vi "MAIN_init_all_global.vi"(1 "error in":errorcluster) -> (0 "error out":errorcluster)   [LabVIEW 2015]
uses:
  GLOBAL/Global_MAIN.vi
  GLOBAL/Global_CAMERA.vi
  GLOBAL/Global_MCL_piezo.vi
  GLOBAL/Global_DAQ.vi
  GLOBAL/Global_ASI_stage.vi
  GLOBAL/Global_ABORT.vi
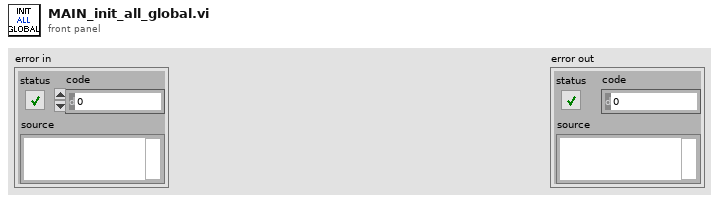
[diagram p1: front panel]
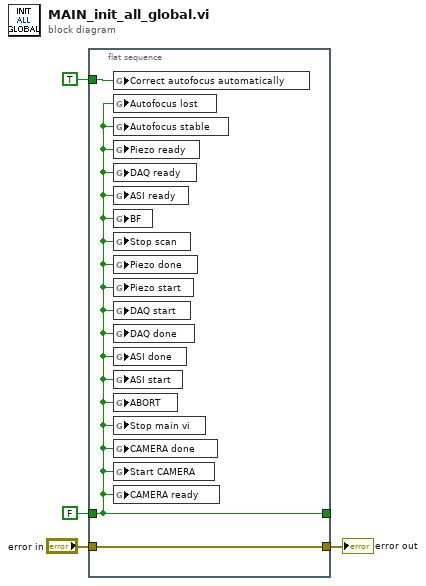
[diagram p0: block diagram]
diagram:
  n1 = flat-sequence {
    tunnel: FALSE ("Stop main vi") -> [w7]
    tunnel: [w7] -> _
    tunnel: "error in" -> [w6]
    tunnel: [w6] -> w2
    tunnel: TRUE ("Stop main vi") -> [w5]
    frame #0 {
      n2 = global write "Global_MAIN.vi" "Correct autofocus automatically"(w5) -> ()
      n3 = global write "Global_MCL_piezo.vi" "Autofocus lost"(w7) -> ()
      n4 = global write "Global_MCL_piezo.vi" "Autofocus stable"(w7) -> ()
      n5 = global write "Global_MCL_piezo.vi" "Piezo ready"(w7) -> ()
      n6 = global write "Global_DAQ.vi" "DAQ ready"(w7) -> ()
      n7 = global write "Global_ASI_stage.vi" "ASI ready"(w7) -> ()
      n8 = global write "Global_ASI_stage.vi" "BF"(w7) -> ()
      n9 = global write "Global_MAIN.vi" "Stop scan"(w7) -> ()
      n10 = global write "Global_MCL_piezo.vi" "Piezo done"(w7) -> ()
      n11 = global write "Global_MCL_piezo.vi" "Piezo start"(w7) -> ()
      n12 = global write "Global_DAQ.vi" "DAQ start"(w7) -> ()
      n13 = global write "Global_DAQ.vi" "DAQ done"(w7) -> ()
      n14 = global write "Global_ASI_stage.vi" "ASI done"(w7) -> ()
      n15 = global write "Global_ASI_stage.vi" "ASI start"(w7) -> ()
      n16 = global write "Global_ABORT.vi" "ABORT"(w7) -> ()
      n17 = global write "Global_MAIN.vi" "Stop main vi"(w7) -> ()
      n18 = global write "Global_CAMERA.vi" "CAMERA done"(w7) -> ()
      n19 = global write "Global_CAMERA.vi" "Start CAMERA"(w7) -> ()
      n20 = global write "Global_CAMERA.vi" "CAMERA ready"(w7) -> ()
    }
  }
  "error out" <- w2
